vi "Register Execution.vi"(0 "Engine in":refnum<class "Engine.lvclass">, 7 "Execution":T1, 11 "error in (no error)":errorcluster) -> (4 "Engine out":refnum<class "Engine.lvclass">, 15 "error out":errorcluster)   [LabVIEW 2019, in "HTS.lvlib" / "Engine.lvclass"]
uses:
  Engine.lvclass
  Execution/Execution.lvclass
  Execution/Typedefs/Session Handle.ctl
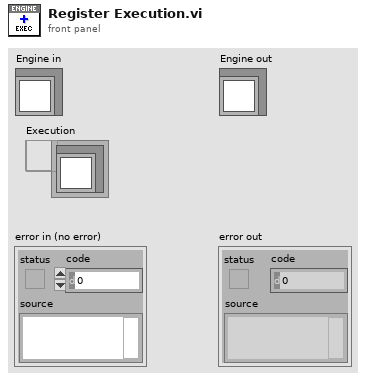
[diagram p1: front panel]
types:
  T1 = typedef "HTS.lvlib/Execution.lvclass/Session Handle.ctl" = refnum<data-value>
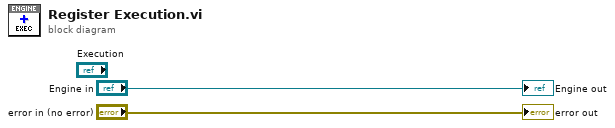
[diagram p0: block diagram]
diagram:
  "error out" <- "error in (no error)"
  "Engine out" <- "Engine in"
